vi "Query with 1D Integer Result.vi"(8 "error in (no error)":errorcluster, 10 "Query string":string, 11 "mysql in":refnum<class "mysql.lvclass">) -> (0 "error out":errorcluster, 2 "Result":i32[](array[numeric]), 3 "mysql out":refnum<class "mysql.lvclass">)   [LabVIEW 2020, in "mysql.lvlib" / "mysql.lvclass"]
uses:
  mysql.lvclass
  d067ab02-a97b-4b6d-9667-43caa71c41f2.vi
  d067ab02-a97b-4b6d-9667-43caa71c41f2.vi/b907deff-c37a-44c2-a9ed-731a17cc9209.vi
  d067ab02-a97b-4b6d-9667-43caa71c41f2.vi/afff7b20-c7b0-42fc-a243-897f31e77240.vi
  private/Mysql command.vi
  private/Mysql data reader 1D integer.vi
  private/ping connection and reopen if needed.vi
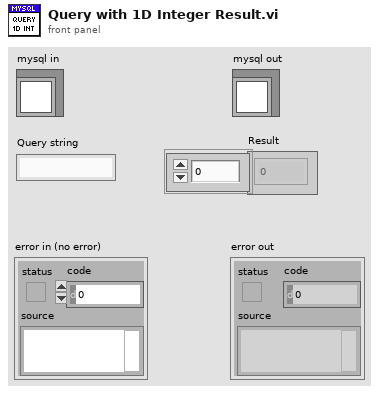
[diagram p1: front panel]
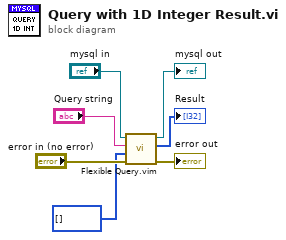
[diagram p0: block diagram]
diagram:
  n1 = call "Flexible Query.vim"("error in (no error)"="error in (no error)", "Type in"=i32[] [] ("Result 2"), "Query string"="Query string", "mysql in"="mysql in") -> ("error out"=→"error out":errorcluster, "Result"=→"Result":i32[], "mysql out"=→"mysql out":refnum<class "mysql.lvclass">)  [unwired: 5 in]
